vi "Load App.vi"(8 "Error In":errorcluster, 9 "Open Actor Core front panel? (F)":bool, 10 "Application Controller.lvclass":refnum<class "Application Controller.lvclass">, 11 "Status Notifier":refnum<notifier>) -> (0 "Error Out":errorcluster)   [LabVIEW 2018, in "Application Controller.lvclass"]
uses:
  Application Controller.lvclass
  C:/github/LabActor/Template Module/Template Module.lvclass
  C:/Program Files/National Instruments/LabVIEW 2018/vi.lib/ActorFramework/Actor/Actor.lvclass
  Template Module/Template Module.lvclass/Template Module.ctl
  Application Controller.lvclass/Application Controller.ctl
  Template Module/Write Name.vi
  Write Launch Notifier.vi
  Write Start-up configuration file.vi
  <vilib>/ActorFramework/Actor/Actor.lvclass
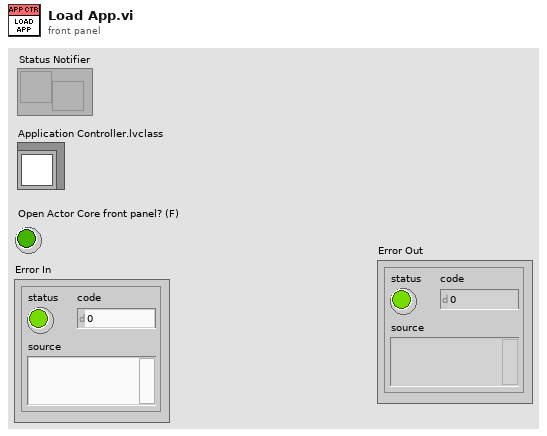
[diagram p1: front panel]
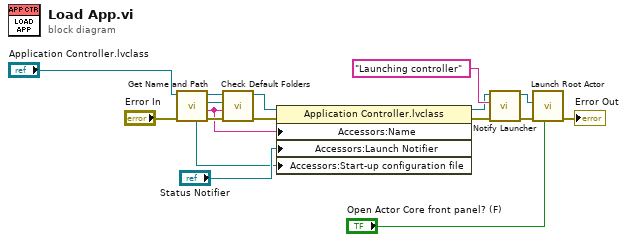
[diagram p0: block diagram]
diagram:
  n1 = call-dynamic "Get Name and Path.vi"("error in (no error)"="Error In", "Application Controller in"="Application Controller.lvclass") -> ("error out"=w4:errorcluster, "Name"=w1:string, "Application folder"=w2:path, "Application Controller out"=w6:refnum<class "Application Controller.lvclass">, "Start-up configuration path"=w7:path)  [unwired: 5 in]
  n2 = call-dynamic "Check Default Folders.vi"("error in (no error)"=w4, "Application name"=w1, "Application folder"=w2, "Application Controller in"=w6) -> ("error out"=w3:errorcluster, "Application Controller out"=w5:refnum<class "Application Controller.lvclass">)  [unwired: 6 in]
  n3 = property class="Application Controller.lvclass"(reference=w5, error in=w3, "Accessors:Name"=w1, "Accessors:Launch Notifier"="Status Notifier", "Accessors:Start-up configuration file"=w7) -> (reference out=w10:refnum<class "Application Controller.lvclass">, error out=w12:errorcluster)
  n4 = call-dynamic "Notify Launcher.vi"("error in (no error)"=w12, "Notification"="Launching controller" ("notification"), "Application Controller in"=w10) -> ("error out"=w15:errorcluster, "Application Controller out"=w16:refnum<class "Application Controller.lvclass">)  [unwired: 7 in]
  n5 = call <vilib>:"Launch Root Actor.vi"("Open Actor Core front panel? (F)"="Open Actor Core front panel? (F)", "error in (no error)"=w15, "Actor"=w16) -> ("error out"=→"Error Out":errorcluster)  [unwired: 7 in, 1 out]
